vi "Get Master DG.vi"(8 "error in (no error)":errorcluster, 11 "BME_DG_System in":refnum<class "BME_DG_System.lvclass">) -> (0 "error out":errorcluster, 2 "BME_DG_Base.lvclass":refnum<class "BME_DG_Base.lvclass">, 3 "BME_DG_System out":refnum<class "BME_DG_System.lvclass">)   [LabVIEW 2009, in "POLARIS BME DG.lvlib" / "BME_DG_System.lvclass"]
uses:
  BME_DG_System.lvclass
  BME_DG_Base/BME_DG_Base.lvclass
  BME_DG_System.lvclass/BME_DG_System.ctl
  POLARIS BME DG.lvlib
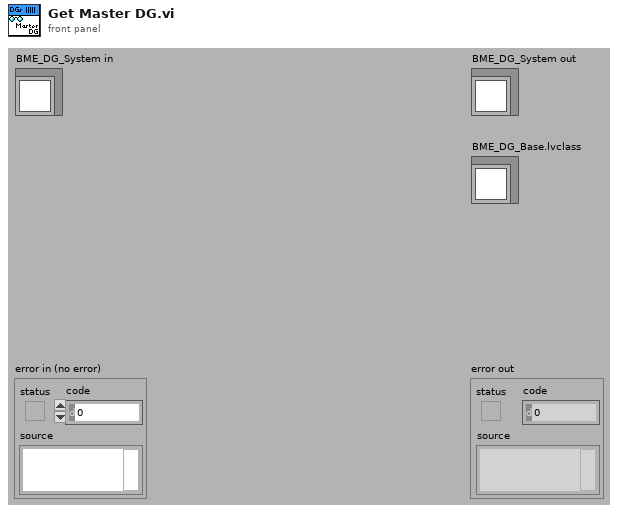
[diagram p1: front panel]
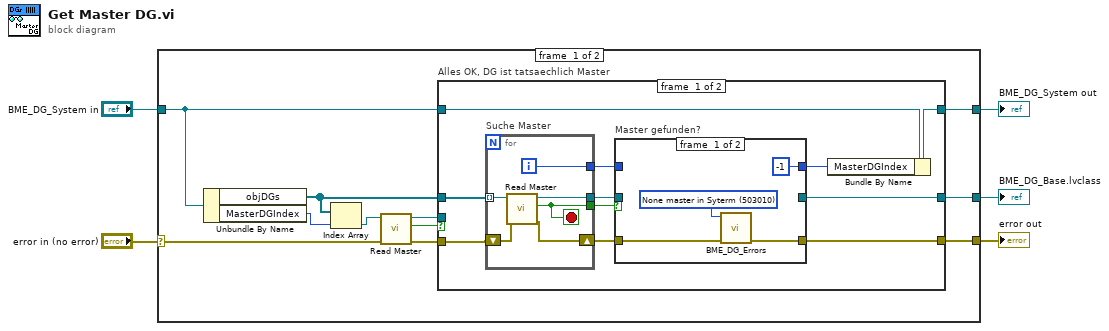
[diagram p0: block diagram]
diagram:
  n1 = case shown="No Error" "error in (no error)" {
    selector: "error in (no error)" -> [w7 w44]
    tunnel: [w6 w44] -> w4
    tunnel: [w9 w45] -> w2
    tunnel: "BME_DG_System in" -> [w10 w45]
    tunnel: [w12 _] -> w1
    frame #0 {
      n2 = Unbundle By Name(w10) -> ("objDGs"=w11:refnum<class "BME_DG_Base.lvclass">[], "MasterDGIndex"=w16:i32)
      n3 = Index Array(array=w11, index=w16) -> (element=w15:refnum<class "BME_DG_Base.lvclass">)
      n4 = call-dynamic "Read Master.vi"("error in (no error)"=w7, "BME_DG_Base in"=w15) -> ("error out"=w8:errorcluster, "Master?"=w14:bool, "BME_DG_Base out"=w13:refnum<class "BME_DG_Base.lvclass">)  [unwired: 6 in, 1 out]
      n5 = case "Alles OK, DG ist tatsaechlich Master" shown="False" w14 {
        tunnel: w13 -> [_ w43]
        tunnel: [w20 w43] -> w12
        tunnel: w11 -> [w27 _]
        tunnel: w10 -> [w26 w42]
        tunnel: [w25 w42] -> w9
        tunnel: w8 -> [w23 w41]
        tunnel: [w19 w41] -> w6
        frame #0 {
          n6 = for "Suche Master" {
            tunnel: w27 -> [w40] mode=indexing
            tunnel: [w39] -> w21
            tunnel: [w38] -> w18
            tunnel: [w37] -> w24
            shift-right: [w35] -> w22
            shift-left: w23 -> [w36]
            i -> [w38]
            stop <- w37 stop-if-true
            n7 = call-dynamic "Read Master.vi"("error in (no error)"=w36, "BME_DG_Base in"=w40) -> ("error out"=w35:errorcluster, "Master?"=w37:bool, "BME_DG_Base out"=w39:refnum<class "BME_DG_Base.lvclass">)  [unwired: 6 in, 1 out]
          }
          n8 = case "Master gefunden?" shown="False" w24 {
            tunnel: w22 -> [w31 w33]
            tunnel: [_ w34] -> w20
            tunnel: w21 -> [_ w34]
            tunnel: [w29 w33] -> w19
            tunnel: w18 -> [_ w32]
            tunnel: [-1 w32] -> w17
            frame #0 {
              w30 = 503010 items=["Channel refers itself"=503001, "Deadloop"=503002, "Negative Delay"=503003, "Delay Card not found"=503004, "Channel not found"=503005, "Parse Error"=503006, "Not Supported"=503007, "Systen not found"=503008, "To much masters"=503009, "None master in Syterm"=503010, "InterruptError"=503011, "ChnlPeriodeWarning"=503012] ("error")
              n9 = call "BME_DG_Errors.vi"("error in (no error)"=w31, "error"=w30) -> ("error out"=w29:errorcluster)  [unwired: 9 in]
            }
            frame #1 {
            }
          }
          n10 = Bundle By Name(cluster=w26, "MasterDGIndex"=w17) -> (w25:refnum<class "BME_DG_System.lvclass">)
        }
        frame #1 {
        }
      }
    }
    frame #1 {
    }
  }
  "error out" <- w4
  "BME_DG_System out" <- w2
  "BME_DG_Base.lvclass" <- w1
